vi "Для калибровки АЧТ.vi"() -> ()   [LabVIEW 2018]
panel:
  out "Time, с":dbl
  out "0.0_cur, A":dbl caption="measurement" format="%_6g"
  out "0.1_cur, A":dbl caption="measurement" format="%_6g"
  out "1.0_cur, A":dbl caption="measurement" format="%_6g"
  out "1.1_cur, A":dbl caption="measurement" format="%_6g"
  in  "Result":path=path "C:/Users/agest/Downloads/Telegram Desktop"
  in  "Папка":path=path "C:/Users/agest/Downloads/Telegram Desktop/ABD"
  # "В папке с логами АЧТ не должно быть ничего лишнего"
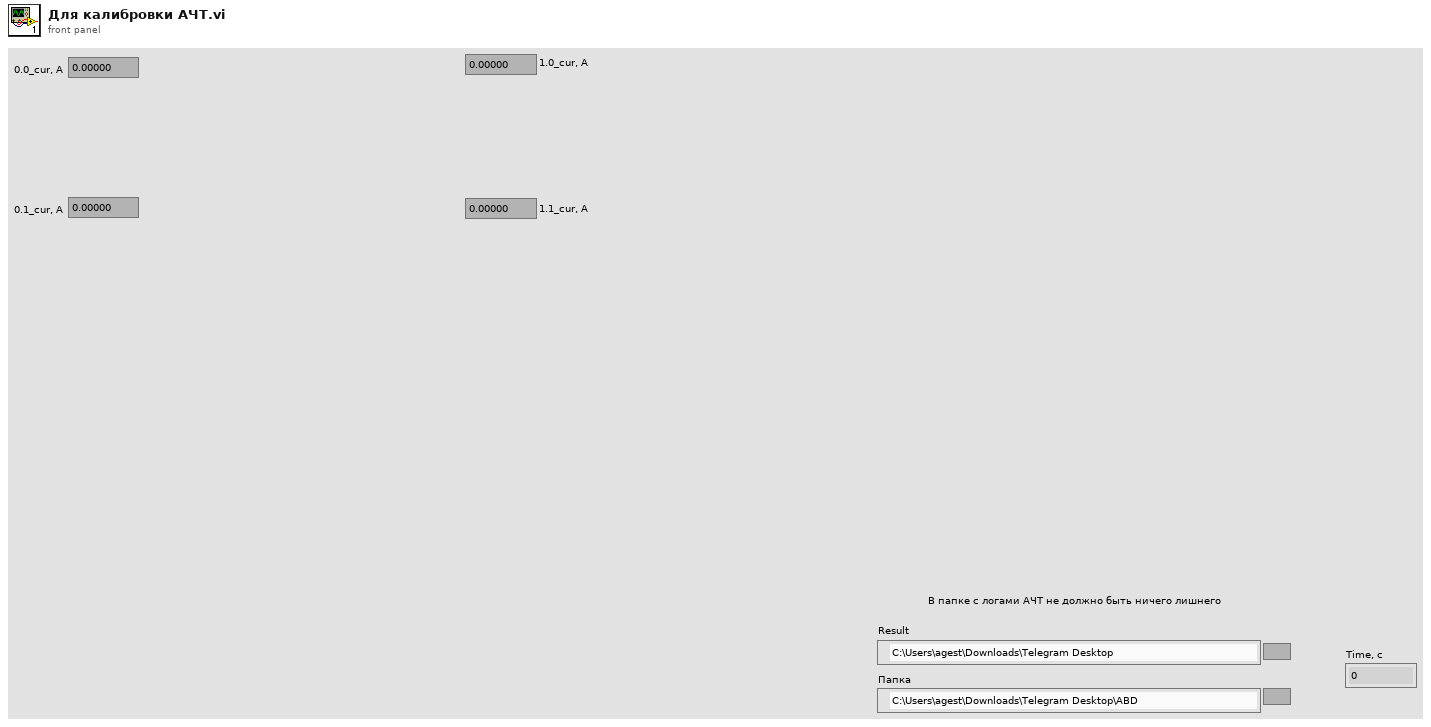
[diagram p1: front panel]
types:
  T1 = enum16{"open", "replace", "create", "open or create", "replace or create", "replace or create with confirmation"}
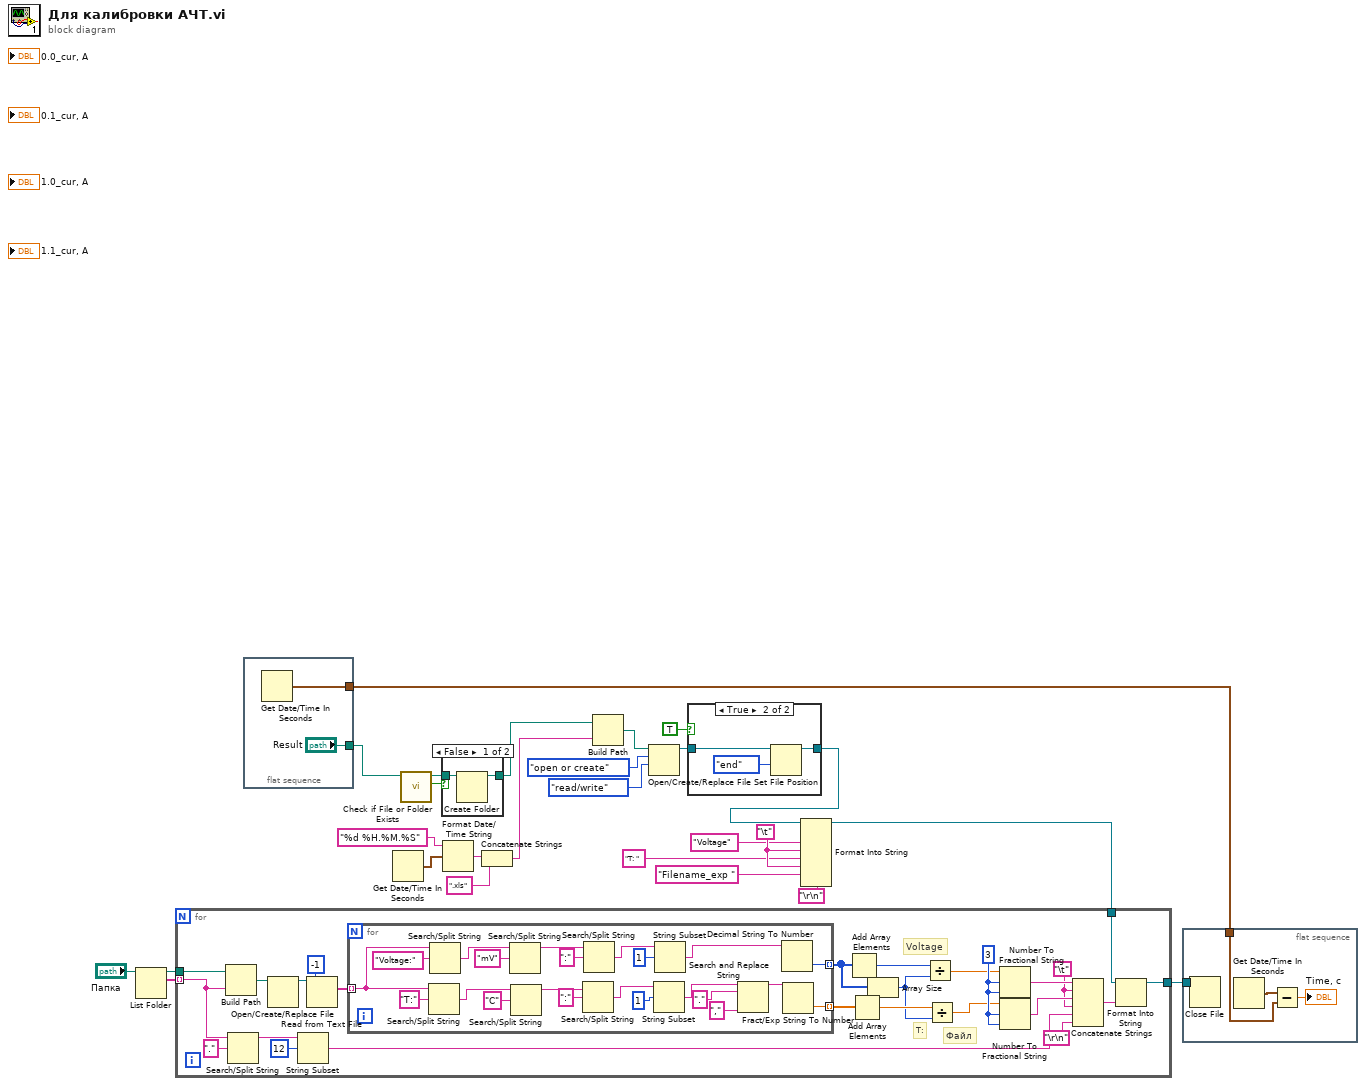
[diagram p0: block diagram]
diagram:
  w23 = "\t"
  n1 = List Folder(path="Папка") -> (path out=w25:path, filenames=w24:string[])  [unwired: 3 in, 2 out]
  n2 = flat-sequence {
    tunnel: ["Result"] -> w5
    tunnel: [w27] -> w1
    frame #0 {
      n3 = Get Date/Time In Seconds() -> (seconds since 1Jan1904=w27:timestamp)
    }
  }
  n4 = Get Date/Time In Seconds() -> (seconds since 1Jan1904=w12:timestamp)
  n5 = call <vilib>:"Check if File or Folder Exists.vi"("path"=w5) -> ("file or folder exists?"=w7:bool, "dup path"=w6:path)  [unwired: 8 in, 1 out]
  n6 = case shown="False" w7 {
    tunnel: w6 -> [w30 w31]
    tunnel: [w29 w31] -> w19
    frame False {
      n7 = Create Folder(path (use dialog)=w30) -> (created path=w29:path)  [unwired: 2 in, 2 out]
    }
    frame True {
    }
  }
  n8 = Format Date/Time String(time format string (%c)="%d %H.%M.%S", seconds (now)=w12) -> (date/time string=w15:string)  [unwired: 1 in]
  n9 = Concatenate Strings(w15, ".xls" ("string")) -> (w17:string)
  n10 = Build Path(base path=w19, name or relative path=w17) -> (appended path=w14:path)
  n11 = Open/Create/Replace File(file path (use dialog)=w14, operation (0:open)=T1."open or create", access (0:read/write)=enum16{"read/write", "read-only", "write-only"}."read/write") -> (refnum out=w11:refnum<file>)  [unwired: 3 in, 2 out]
  n12 = case shown="True" TRUE {
    tunnel: w11 -> [w32 w35]
    tunnel: [w32 w33] -> w18
    frame False {
    }
    frame True {
      n13 = Set File Position(refnum=w35, from (0:start)=enum16{"start", "end", "current"}."end") -> (refnum out=w33:refnum<file>)  [unwired: 2 in, 1 out]
    }
  }
  n14 = Format Into String(initial string=w18, "Voltage" ("input 1"), w23, "T: " ("input 1"), w23, "Filename_exp " ("input 1"), "\r\n") -> (resulting string=w3:refnum<file>)  [unwired: 2 in, 1 out]
  n15 = for {
    tunnel: w25 -> [w53]
    tunnel: w24 -> [w50] mode=indexing
    tunnel: w3 -> [w38]
    tunnel: [w37] -> w2
    w43 = i16 3 ("width (-)")
    w42 = "\t"
    # "T:"
    # "Voltage"
    # "Файл"
    n16 = Build Path(base path=w53, name or relative path=w50) -> (appended path=w52:path)
    n17 = Search/Split String(string=w50, search string/char (-)=".") -> (substring before match=w48:string)  [unwired: 1 in, 2 out]
    n18 = Open/Create/Replace File(file path (use dialog)=w52) -> (refnum out=w51:refnum<file>)  [unwired: 5 in, 2 out]
    n19 = String Subset(string=w48, offset (0)=12) -> (substring=w39:string)  [unwired: 1 in]
    n20 = Read from Text File(file (use dialog)=w51, count=-1) -> (text=w60:string[])  [unwired: 2 in, 3 out]
    n21 = for {
      tunnel: w60 -> [w81] mode=indexing
      tunnel: [w66] -> w57 mode=indexing
      tunnel: [w65] -> w58 mode=indexing
      n22 = Search/Split String(string=w81, search string/char (-)="T:") -> (match + rest of string=w77:string)  [unwired: 1 in, 2 out]
      n23 = Search/Split String(string=w81, search string/char (-)="Voltage:") -> (match + rest of string=w79:string)  [unwired: 1 in, 2 out]
      n24 = Search/Split String(string=w79, search string/char (-)="mV") -> (substring before match=w75:string)  [unwired: 1 in, 2 out]
      n25 = Search/Split String(string=w77, search string/char (-)="C") -> (substring before match=w74:string)  [unwired: 1 in, 2 out]
      n26 = Search/Split String(string=w74, search string/char (-)=":") -> (match + rest of string=w68:string)  [unwired: 1 in, 2 out]
      n27 = Search/Split String(string=w75, search string/char (-)=":") -> (match + rest of string=w71:string)  [unwired: 1 in, 2 out]
      n28 = String Subset(string=w68, offset (0)=1) -> (substring=w64:string)  [unwired: 1 in]
      n29 = String Subset(string=w71, offset (0)=1) -> (substring=w67:string)  [unwired: 1 in]
      n30 = Search and Replace String(input string=w64, search string=".", replace string="," ("replace string (\"\")")) -> (result string=w61:string)  [unwired: 5 in, 3 out]
      n31 = Decimal String To Number(string=w67) -> (number=w66:i32)  [unwired: 2 in, 1 out]
      n32 = Fract/Exp String To Number(string=w61) -> (number=w65:dbl)  [unwired: 3 in, 1 out]
    }
    n33 = Add Array Elements(numeric array=w57) -> (sum=w56:i32)
    n34 = Add Array Elements(numeric array=w58) -> (sum=w55:dbl)
    n35 = Array Size(array=w57) -> (size(s)=w54:i32)
    n36 = Divide(x=w56, y=w54) -> (x/y=w41:dbl)
    n37 = Divide(x=w55, y=w54) -> (x/y=w40:dbl)
    n38 = Number To Fractional String(number=w41, width (-)=w43, precision (6)=w43) -> (F-format string=w45:string)  [unwired: 1 in]
    n39 = Number To Fractional String(number=w40, width (-)=w43, precision (6)=w43) -> (F-format string=w44:string)  [unwired: 1 in]
    n40 = Concatenate Strings(w45, w42, w44, w42, w39, "\r\n") -> (w46:string)
    n41 = Format Into String(initial string=w38, w46) -> (resulting string=w37:refnum<file>)  [unwired: 2 in, 1 out]
  }
  n42 = flat-sequence {
    tunnel: w2 -> [w86]
    tunnel: w1 -> [w85]
    frame #0 {
      n43 = Close File(refnum=w86) -> ()  [unwired: 1 in, 2 out]
      n44 = Get Date/Time In Seconds() -> (seconds since 1Jan1904=w83:timestamp)
      n45 = Subtract(x=w83, y=w85) -> (x-y=→"Time, с":dbl)
    }
  }
